vi "Read.vi"(8 "error in (no error)":errorcluster, 10 "ReadElements":u32=10000, 11 "AODAcq in":refnum<class "AODAcq.lvclass">) -> (0 "error out":errorcluster, 1 "TemporalData":waveform(dbl)[](array[waveform]), 2 "ImData":waveform(i32)[](array[waveform]), 3 "AODAcq out":refnum<class "AODAcq.lvclass">, 4 "ReadFractionOut":dbl, 5 "MotionData":waveform(i32)[](array[waveform]), 6 "Done":bool, 7 "MotionCorrectionData":waveform(i32)[](array[waveform]))   [LabVIEW 2014, in "AODAcq.lvclass"]
uses:
  AODAcq.lvclass
  FPGA_Control/FPGAState.ctl
  AODAcq.lvclass/AODAcq.ctl
  <vilib>/Utility/error.llb/Error Cluster From Error Code.vi
  <vilib>/rvi/errors/niLvFpgaAdjustHostInterfaceError.vi
  Program Files (x86)/National Instruments/LabVIEW 2014/Targets/NI/FPGA/StockFPGA_IntfPrivate/ScriptTemplates/StockFPGA_PlugInRead32.vi
  <vilib>/rvi/interface/nirviMethod/nirviMethod.xnode
  FPGA_Control/AODRef.ctl
  FPGA Bitfiles/AodScanner_FPGATarget_AODControl(FPGA)_TyJc9yYmyGA.lvbitx
  <vilib>/rvi/interface/nirviReadWriteControl/nirviReadWriteControl.xnode
  NiFpgaLv.dll
  <vilib>/FPGAPlugInAG/PXIe-7965R/niLvFpga_Read32_PXIe-7965R.vi
  <vilib>/rvi/interface/nirviReadWriteControl/niFpgaRWControlAccessTimeoutTemplate.vi
  <vilib>/FPGAPlugInAG/PXIe-7965R/niLvFpga_ReadFifo_PXIe-7965R.vi
  <vilib>/rvi/errors/niLvFpgaMergeErrorWithErrorCode.vi
panel:
  out "PMT Transfers":i32
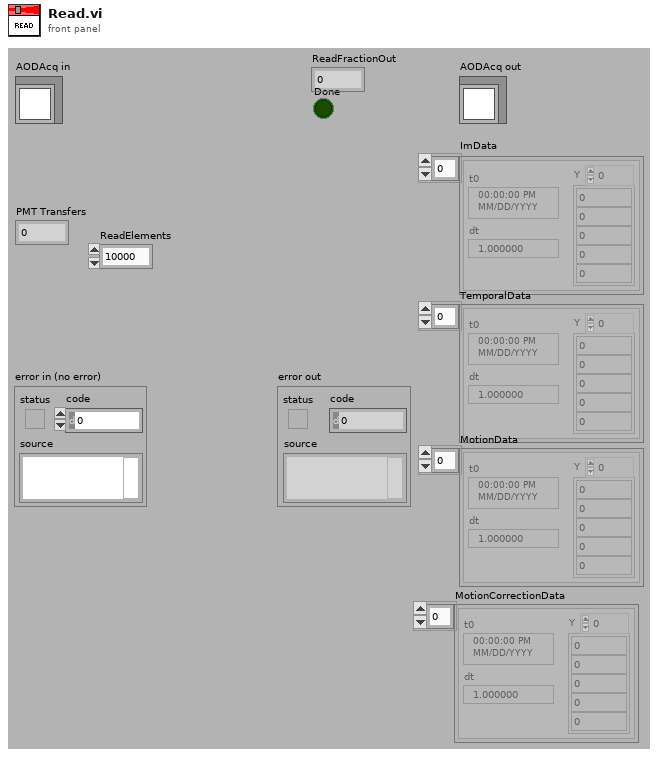
[diagram p1: front panel]
types:
  T1 = typedef "FPGAState.ctl" = enum16{"Idle", "Arm Scan", "Scan", "End Scan"}
  T2 = typedef "AODRef.ctl" = refnum<k20>
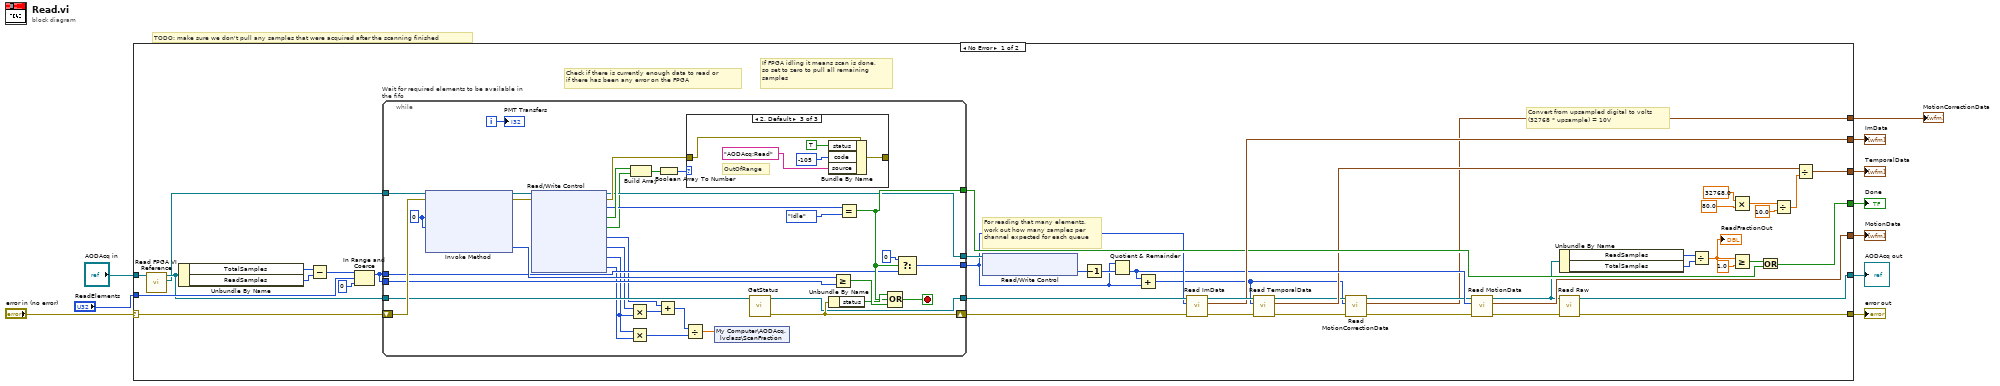
[diagram p0: block diagram]
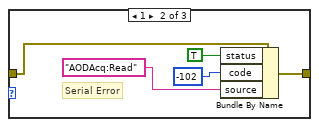
[diagram p3: hidden frame]
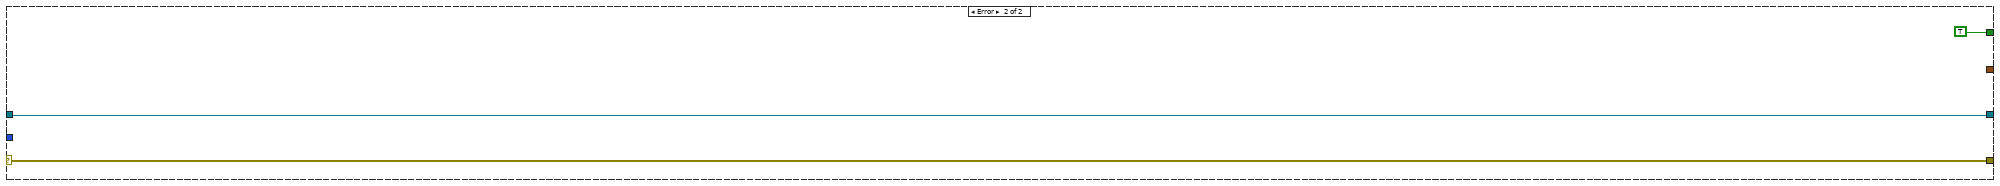
[diagram p4: hidden frame]
diagram:
  # "TODO: make sure we don't pull any samples that were acquired after the scanning finished"
  n1 = case shown="No Error" "error in (no error)" {
    selector: "error in (no error)" -> [w50 w103]
    tunnel: [w17 w103] -> w9
    tunnel: [w19 w102] -> w7
    tunnel: "AODAcq in" -> [w55 w102]
    tunnel: "ReadElements" -> [w52 _]
    tunnel: [w39 _] -> w5
    tunnel: [w28 _] -> w4
    tunnel: [w38 _] -> w3
    tunnel: [w35 TRUE] -> w2
    tunnel: [w14 _] -> w1
    frame No Error {
      # "If FPGA idling it means scan is done, \nso set to zero to pull all remaining\nsamples"
      # "Check if there is currently enough data to read or \nif there has been any error on the FPGA"
      # "Convert from upsampled digital to volts\n(32768 * upsample) = 10V"
      # "For reading that many elements,\nwork out how many samples per\nchannel expected for each queue"
      n2 = call-dynamic "Read FPGA VI Reference.vi"("AODAcq in"=w55) -> ("FPGA VI Reference"=w22:T2, "AODAcq out"=w49:refnum<class "AODAcq.lvclass">)  [unwired: 8 in, 1 out]
      n3 = Unbundle By Name(w49) -> ("TotalSamples"=w51:u64, "ReadSamples"=w44:u64)
      n4 = Subtract(x=w51, y=w44) -> (x-y=w53:u64)
      n5 = In Range and Coerce(upper limit=w53, x=w52, lower limit=u32 0) -> (coerced(x)=w21:u64)  [unwired: 1 out]
      n6 = while "Wait for required elements to be available in the fifo" {
        tunnel: w21 -> [w76]
        tunnel: w22 -> [w88]
        tunnel: [w66] -> w31
        tunnel: [w62] -> w34
        tunnel: w49 -> [w73]
        shift-right: [w71] -> w47
        shift-left: w50 -> [w85]
        tunnel: [w70] -> w45
        tunnel: [w69] -> w36
        tunnel: w21 -> [w67]
        i -> [w86]
        stop <- w87 stop-if-true
        w89 = u32 0 ("Number of Elements")
        n7 = xnode "Invoke Method"("FPGA VI Reference In"=w88, "error in"=w85, "Number of Elements"=w89, "Timeout (ms)"=w89) -> ("FPGA VI Reference Out"=w80:T2, "error out"=w81:errorcluster, "Elements Remaining"=w77:u32)  [unwired: 1 out]
        n8 = xnode "Read/Write Control"("FPGA VI Reference In"=w80, "error in"=w81) -> ("FPGA VI Reference Out"=w62:T2, "error out"=w75:errorcluster, "Status.Sequencer"=w78:T1, "Error.Sequencer"=w84:bool, "Error.OutOfRange"=w56:bool, "Status.PointNum"=w58:u32, "Status.RepNum"=w60:u32, "Scan.NumPoints"=w61:u32, "Scan.NumReps"=w65:i32)
        n9 = Multiply(x=w60, y=w61) -> (x*y=w59:u32)
        n10 = Multiply(x=w61, y=w65) -> (x*y=w64:u32)
        n11 = Build Array(w84, w56) -> (w83:bool[])
        n12 = Add(x=w58, y=w59) -> (x+y=w57:u32)
        n13 = Boolean Array To Number(Boolean array=w83) -> (number=w82:u32)
        n14 = Divide(x=w57, y=w64) -> (x/y=w63:dbl)
        n15 = case shown="2, Default" w82 {
          tunnel: [w90 w92 w97] -> _
          tunnel: w75 -> [w90 w91 w96]
          frame 0 {
          }
          frame 1 {
            # "Serial Error"
            n16 = Bundle By Name(cluster=w91, "status"=TRUE, "code"=-102, "source"="AODAcq:Read") -> (w92:errorcluster)
          }
          frame 2, Default {
            # "OutOfRange"
            n17 = Bundle By Name(cluster=w96, "status"=TRUE, "code"=-105, "source"="AODAcq:Read") -> (w97:errorcluster)
          }
        }
        n18 = shared-variable "My Computer\\AODAcq.lvclass\\ScanFraction"(w63) -> ()  [unwired: 1 in, 1 out]
        n19 = call-dynamic "GetStatus.vi"("AODAcq in"=w73) -> ("error out"=w71:errorcluster, "AODAcq out"=w70:refnum<class "AODAcq.lvclass">)  [unwired: 8 in, 1 out]
        n20 = Unbundle By Name(w71) -> ("status"=w72:bool)
        n21 = Greater Or Equal?(x=w77, y=w76) -> (x >= y?=w74:bool)
        n22 = Equal?(x=w78, y=FPGAState."Idle" ("x")) -> (x = y?=w69:bool)
        n23 = Compound Arithmetic op=OR(w72, w69, w74) -> (w87:bool)
        n24 = Select(t=u64 0, s=w69, f=w67) -> (s? t:f=w66:u64)
        "PMT Transfers" <- w86
      }
      n25 = xnode "Read/Write Control"("FPGA VI Reference In"=w34) -> ("Scan.Motion Increment"=w33:u32)  [unwired: 1 in, 2 out]
      n26 = Decrement(x=w33) -> (x-1=w32:u32)
      n27 = Quotient & Remainder(x=w31, y=w32) -> (floor(x/y)=w30:u64)  [unwired: 1 out]
      n28 = Add(x=w30, y=w31) -> (x+y=w13:u64)
      n29 = call-dynamic "Read ImData.vi"("error in (no error)"=w47, "ReadSize"=w31, "AODAcq in"=w45) -> ("error out"=w46:errorcluster, "ImData"=w39:waveform(i32)[], "AODAcq out"=w48:refnum<class "AODAcq.lvclass">)  [unwired: 6 in]
      n30 = call-dynamic "Read TemporalData.vi"("error in (no error)"=w46, "ReadSize"=w13, "AODAcq in"=w48) -> ("error out"=w12:errorcluster, "TemporalData"=w29:waveform(i32)[], "AODAcq out"=w16:refnum<class "AODAcq.lvclass">)  [unwired: 6 in]
      n31 = call "Read MotionCorrectionData.vi"("error in (no error)"=w12, "ReadSize"=w13, "AODAcq in"=w16) -> ("error out"=w11:errorcluster, "MotionCorrectionData"=w14:waveform(i32)[], "AODAcq out"=w15:refnum<class "AODAcq.lvclass">)  [unwired: 6 in]
      n32 = call-dynamic "Read MotionData.vi"("error in (no error)"=w11, "ReadSize"=w30, "AODAcq in"=w15) -> ("error out"=w18:errorcluster, "MotionData"=w38:waveform(i32)[], "AODAcq out"=w20:refnum<class "AODAcq.lvclass">)  [unwired: 6 in]
      n33 = Unbundle By Name(w20) -> ("ReadSamples"=w43:u64, "TotalSamples"=w42:u64)
      n34 = call-dynamic "Read Raw.vi"("error in (no error)"=w18, "AODAcq in"=w20) -> ("error out"=w17:errorcluster, "AODAcq out"=w19:refnum<class "AODAcq.lvclass">)  [unwired: 8 in]
      n35 = Divide(x=w43, y=w42) -> (x/y=w41:dbl)
      "ReadFractionOut" <- w41
      n36 = Multiply(x=32768.0, y=80.0) -> (x*y=w25:dbl)
      n37 = Greater Or Equal?(x=w41, y=1.0) -> (x >= y?=w37:bool)
      n38 = Or(x=w37, y=w36) -> (x .or. y?=w35:bool)
      n39 = Divide(x=w25, y=10.0) -> (x/y=w23:dbl)
      n40 = Divide(x=w29, y=w23) -> (x/y=w28:waveform(dbl)[])
    }
    frame Error {
    }
  }
  "error out" <- w9
  "AODAcq out" <- w7
  "ImData" <- w5
  "TemporalData" <- w4
  "MotionData" <- w3
  "Done" <- w2
  "MotionCorrectionData" <- w1
